vi "Initialize.vi"(6 "Motor Index":u8, 7 "Motor IO Refnum":T1={"SEN"="A/AO0", "PWM"="A/PWM0", "SIGN (Vel Dir)"="A/DIO0", "Enc"="A/ENC", "Generic FPGA Reference"=refnum, "SON"="A/DIO0"}, 8 "error in (no error)":errorcluster, 9 "PID Paras":T3={"Output Range(deg/s)"={"output high"=720.0, "output low"=-720.0}, "PID gains"={"proportional gain (Kc)"=6.5, "integral time (Ti, min)"=0.0075, "derivative time (Td, min)"=0.0005}} {"PID gains"."derivative time (Td, min)" format="%.4f"; "PID gains"."integral time (Ti, min)" format="%.4f"; "PID gains"."proportional gain (Kc)" format="%.4f"; "Output Range(deg/s)"."output low" format="%.2f"; "Output Range(deg/s)"."output high" format="%.2f"}, 10 "Pos Ctrl Paras":T4={"Tolerance(deg)"=0.5, "Loop Time(ms)"=10, "Min Frequency(hz)"=40.0} {"Min Frequency(hz)" format="%#_13g"}, 11 "Servo Drive and  Motor Paras":T5={"Encoder Output Pulses"=900.0, "Gear Ratio(Numerator)"=1000.0, "Gear Ratio(Denominator)"=1.0, "Reduction Ratio"=1.0} {"Gear Ratio(Denominator)" format="%#_10g"}) -> (0 "error out":errorcluster, 3 "SGDV_Ctrl_Class out":refnum<class "SGDV_Ctrl_Class.lvclass">)   [LabVIEW 2013, in "SGDV_Ctrl_v13_lib.lvlib" / "SGDV_Ctrl_Class.lvclass"]
uses:
  SGDV_Ctrl_Class.lvclass
  Controls and General VIs/Servo Drive and  Motor Paras.ctl
  Controls and General VIs/Pos Ctrl Paras.ctl
  Controls and General VIs/PID Paras.ctl
  Controls and General VIs/Motor IO Refnum.ctl
  <vilib>/myRIO/Common/Instrument Driver Framework/Utilities/typedefs/Generic FPGA Reference.ctl
  Controls and General VIs/Motor Coefficients.ctl
  SGDV_Ctrl_Class.lvclass/SGDV_Ctrl_Class.ctl
  SGDV_Ctrl_v13_lib.lvlib
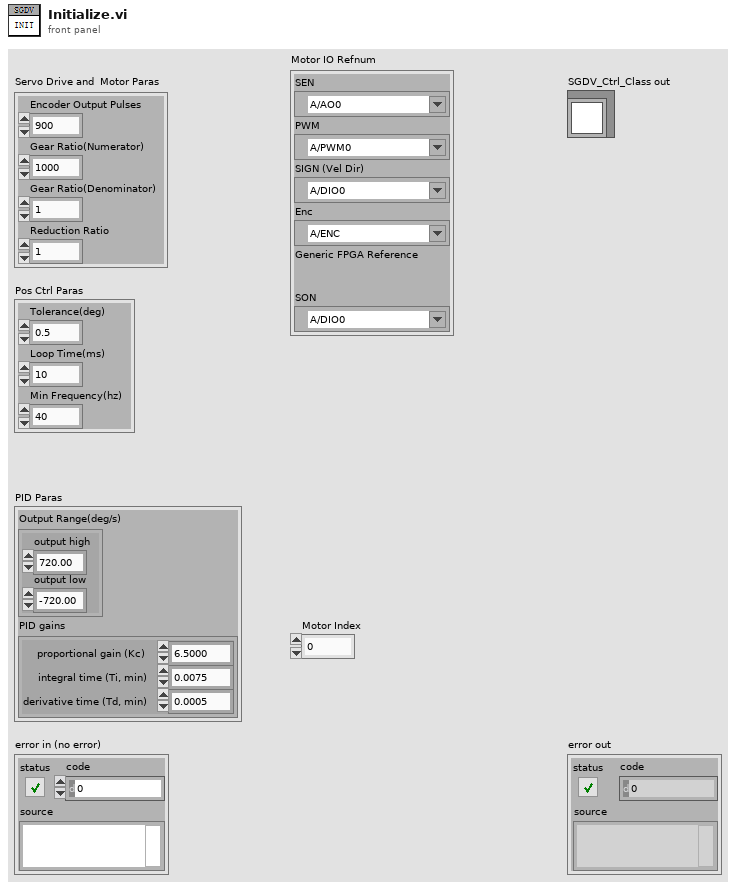
[diagram p1: front panel]
types:
  T1 = typedef "SGDV_Ctrl_v13_lib.lvlib/Motor IO Refnum.ctl" = cluster{"SEN":tag, "PWM":tag, "SIGN (Vel Dir)":tag, "Enc":tag, "Generic FPGA Reference":T2, "SON":tag}
  T2 = typedef "Generic FPGA Reference.ctl" = refnum<k20>
  T3 = typedef "SGDV_Ctrl_v13_lib.lvlib/PID Paras.ctl" = cluster{"Output Range(deg/s)":cluster{"output high":dbl, "output low":dbl}, "PID gains":cluster{"proportional gain (Kc)":dbl, "integral time (Ti, min)":dbl, "derivative time (Td, min)":dbl}}
  T4 = typedef "SGDV_Ctrl_v13_lib.lvlib/Pos Ctrl Paras.ctl" = cluster{"Tolerance(deg)":dbl, "Loop Time(ms)":u32, "Min Frequency(hz)":dbl}
  T5 = typedef "SGDV_Ctrl_v13_lib.lvlib/Servo Drive and  Motor Paras.ctl" = cluster{"Encoder Output Pulses":dbl, "Gear Ratio(Numerator)":dbl, "Gear Ratio(Denominator)":dbl, "Reduction Ratio":dbl}
  T6 = typedef "SGDV_Ctrl_v13_lib.lvlib/Motor Coefficients.ctl" = cluster{"Vel-Coefficient":dbl, "Enc-Coefficient":dbl, "Reduction-Ratio":dbl}
  T7 = typedef "SGDV_Ctrl_v13_lib.lvlib/Init Motor Data.ctl" = cluster{"Init Rev Num":i32, "Init Pul Num":i32, "Init-Motor-Pos(deg)":dbl}
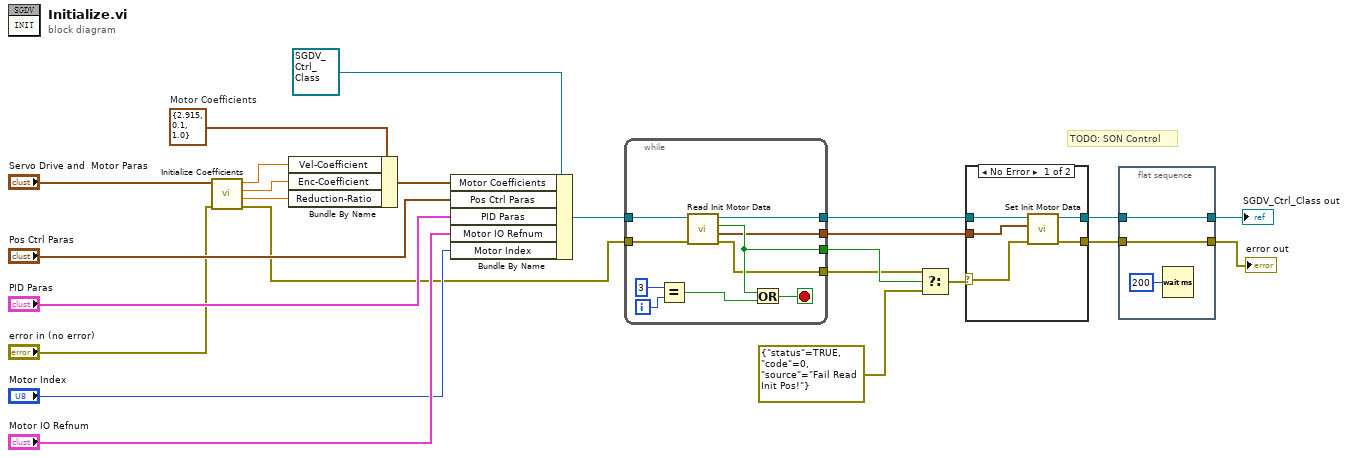
[diagram p0: block diagram]
diagram:
  w23 = T6 {"Vel-Coefficient"=2.915, "Enc-Coefficient"=0.1, "Reduction-Ratio"=1.0}  # Motor Coefficients
  # "TODO: SON Control"
  n1 = call "Initialize Coefficients.vi"("error in (no error)"="error in (no error)", "Servo Drive and  Motor Paras"="Servo Drive and  Motor Paras") -> ("error out"=w11:errorcluster, "Reduction Ratio"=w20:dbl, "Enc-Coefficient"=w21:dbl, "Vel-Coefficient"=w22:dbl)  [unwired: 6 in]
  n2 = Bundle By Name(cluster=w23, "Vel-Coefficient"=w22, "Enc-Coefficient"=w21, "Reduction-Ratio"=w20) -> (w18:T6)
  n3 = Bundle By Name(cluster=refnum<class "SGDV_Ctrl_Class.lvclass"> refnum ("SGDV_Ctrl_v14.2_lib.lvlib:SGDV_Ctrl_Class.lvclass"), "Motor Coefficients"=w18, "Pos Ctrl Paras"="Pos Ctrl Paras", "PID Paras"="PID Paras", "Motor IO Refnum"="Motor IO Refnum", "Motor Index"="Motor Index") -> (w12:refnum<class "SGDV_Ctrl_Class.lvclass">)
  n4 = while {
    tunnel: [w30] -> w6
    tunnel: [w29] -> w10
    tunnel: w12 -> [w28]
    tunnel: w11 -> [w27]
    tunnel: [w26] -> w5
    tunnel: [w25] -> w9
    i -> [w34]
    stop <- w31 stop-if-true
    n5 = Equal?(x=3, y=w34) -> (x = y?=w32:bool)
    n6 = call "Read Init Motor Data.vi"("error in (no error)"=w27, "SGDV_Ctrl_Class in"=w28) -> ("error out"=w25:errorcluster, "Init Motor Data"=w26:T7, "Get Serial Data?"=w29:bool, "SGDV_Ctrl_Class out"=w30:refnum<class "SGDV_Ctrl_Class.lvclass">)  [unwired: 6 in]
    n7 = Or(x=w29, y=w32) -> (x .or. y?=w31:bool)
  }
  n8 = Select(t=w9, s=w10, f=errorcluster {"status"=TRUE, "code"=0, "source"="Fail Read Init Pos!"}) -> (s? t:f=w7:errorcluster)
  n9 = case shown="No Error" w7 {
    selector: w7 -> [w37 w40]
    tunnel: w6 -> [w39 w41]
    tunnel: w5 -> [w38 _]
    tunnel: [w36 w41] -> w4
    tunnel: [w35 w40] -> w3
    frame No Error {
      n10 = call "Set Init Motor Data.vi"("error in (no error)"=w37, "Init Motor Data"=w38, "SGDV_Ctrl_Class in"=w39) -> ("error out"=w35:errorcluster, "SGDV_Ctrl_Class out"=w36:refnum<class "SGDV_Ctrl_Class.lvclass">)  [unwired: 7 in]
    }
    frame Error {
    }
  }
  n11 = flat-sequence {
    tunnel: w4 -> [w44]
    tunnel: [w44] -> w1
    tunnel: w3 -> [w43]
    tunnel: [w43] -> w2
    frame #0 {
      n12 = Wait (ms)(milliseconds to wait=u32 200) -> ()  [unwired: 1 out]
    }
  }
  "SGDV_Ctrl_Class out" <- w1
  "error out" <- w2
